vi "CreateMixtureString.vi"(9 "Odor Mixtures":bool[](array[boolean]), 10 "Concentrations":string[](array[string]), 11 "Odors":string[](array[string])) -> (3 "Odor Mixture String":string)   [LabVIEW 2016]
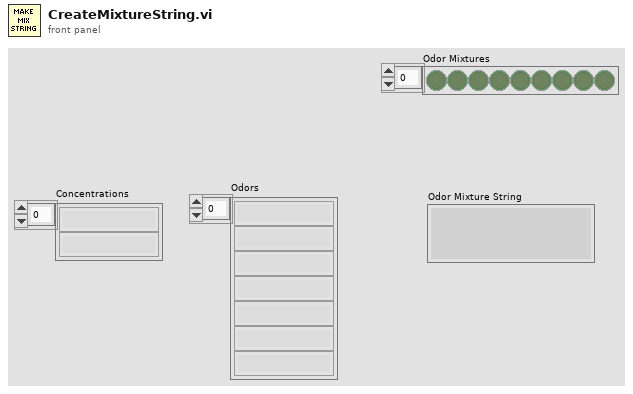
[diagram p1: front panel]
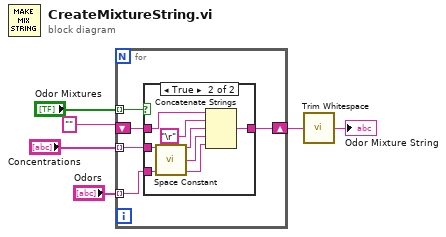
[diagram p0: block diagram]
diagram:
  n1 = for {
    tunnel: "Odors" -> [w11] mode=indexing
    tunnel: "Concentrations" -> [w10] mode=indexing
    tunnel: "Odor Mixtures" -> [w9] mode=indexing
    shift-right: [w7] -> w3
    shift-left: "" -> [w8]
    n2 = case shown="True" w9 {
      tunnel: w11 -> [_ w17]
      tunnel: w10 -> [_ w16]
      tunnel: [w12 w13] -> w7
      tunnel: w8 -> [w12 w14]
      frame False {
      }
      frame True {
        n3 = call <vilib>:"Space Constant.vi"() -> ("String"=w18:string)
        n4 = Concatenate Strings(w14, "\r", w16, w18, w17) -> (w13:string)
      }
    }
  }
  n5 = call <vilib>:"Trim Whitespace.vi"("string"=w3) -> ("trimmed string"=→"Odor Mixture String":string)  [unwired: 1 in]
